vi "Arduino_I2CRead1.vi"() -> ()   [LabVIEW 2019]
uses:
  <vilib>/LabVIEW Interface for Arduino/LabVIEW Interface for Arduino.lvlib
  <vilib>/LabVIEW Interface for Arduino/Type Defs/Connection Type.ctl
  <vilib>/LabVIEW Interface for Arduino/Type Defs/Board Type.ctl
panel:
  out "Erro I2C Write":errorcluster
  out "error out":errorcluster
  out "I2C Data":u8[](array[numeric])
  out "?":dbl
  out "Signal":waveform(dbl)(graph)
  in  "Stopp":bool
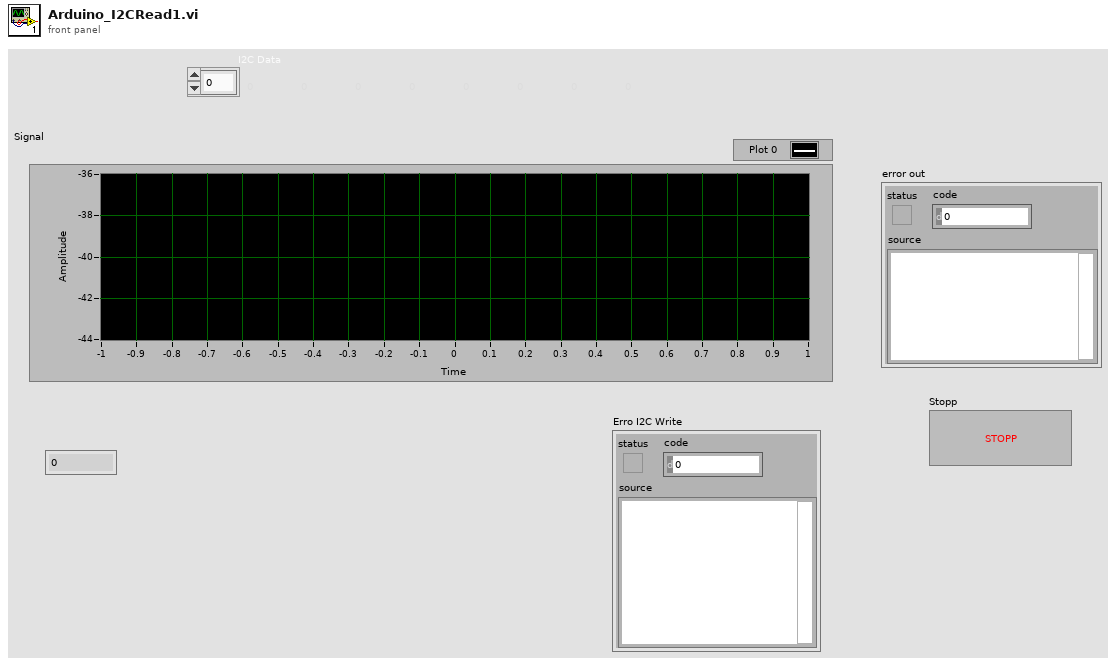
[diagram p1: front panel]
types:
  T1 = typedef "LabVIEW Interface for Arduino.lvlib/Board Type.ctl" = enum16{"Uno", "Dimuelanove w/Atmega 328", "Mega 2560"}
  T2 = typedef "LabVIEW Interface for Arduino.lvlib/Connection Type.ctl" = enum8{"USB / Serial", "XBEE", "BlueSmirf (Bluetooth)"}
  T3 = typedef "LabVIEW Interface for Arduino.lvlib/Arduino Resource.ctl" = cluster{"VISA resource":refnum<visa-resource-name>, "Board Type":T1, "Connection Type":enum8{"USB / Serial"}, "Bytes Per Packet (15)":u8}
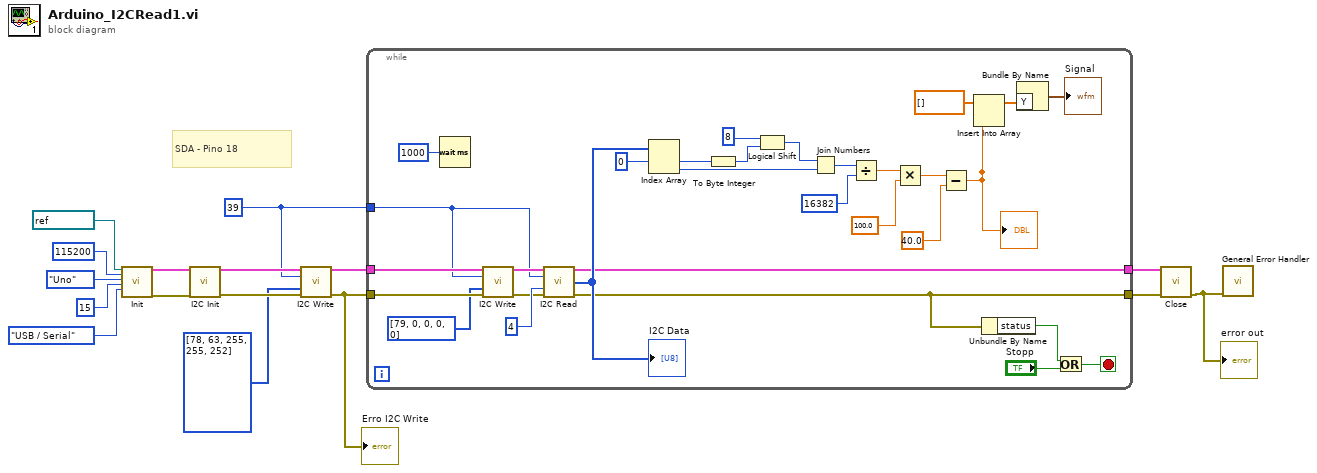
[diagram p0: block diagram]
diagram:
  w3 = u8 39 ("Address (0)")
  # "SDA - Pino 18"
  n1 = call <vilib>:"Init.vi"("VISA resource"=refnum<visa-resource-name> "COM3", "Baud Rate (115200)"=u32 115200, "Board Type (Uno)"=Board_Type."Uno", "Bytes Per Packet (15)"=u32 15, "Connection Type (USB/Serial)"=Connection_Type."USB / Serial") -> ("Arduino Resource"=w16:T3, "error out"=w15:errorcluster)  [unwired: 13 in]
  n2 = call <vilib>:"I2C Init.vi"("Arduino Resource"=w16, "error in"=w15) -> ("Arduino Resource"=w6:T3, "error out"=w4:errorcluster)  [unwired: 12 in]
  n3 = call <vilib>:"I2C Write.vi"("Arduino Resource"=w6, "Address (0)"=w3, "I2C Data Bytes"=u8[] [78, 63, 255, 255, 252] ("Data"), "error in"=w4) -> ("Arduino Resource"=w5:T3, "error out"=w1:errorcluster)  [unwired: 10 in]
  "Erro I2C Write" <- w1
  n4 = while {
    tunnel: w5 -> [w32]
    tunnel: w1 -> [w29]
    tunnel: [w24] -> w9
    tunnel: [w33] -> w7
    tunnel: w3 -> [w27]
    stop <- w41 stop-if-true
    n5 = Wait (ms)(milliseconds to wait=u32 1000 ("Zu wartende ms")) -> ()  [unwired: 1 out]
    n6 = call <vilib>:"I2C Write.vi"("Arduino Resource"=w32, "Address (0)"=w27, "I2C Data Bytes"=u8[] [79, 0, 0, 0, 0] ("Data"), "error in"=w29) -> ("Arduino Resource"=w31:T3, "error out"=w30:errorcluster)  [unwired: 10 in]
    n7 = call <vilib>:"I2C Read.vi"("Arduino Resource"=w31, "Address (0)"=w27, "Bytes To Read"=u8 4, "error in"=w30) -> ("Arduino Resource"=w33:T3, "I2C Data"=w40:u8[], "error out"=w24:errorcluster)  [unwired: 9 in]
    "I2C Data" <- w40
    n8 = Index Array(array=w40, index #1=0 ("Index")) -> (element #1=w23:u8, element #2=w21:u8)  [unwired: 1 in]
    n9 = To Byte Integer(number=w23) -> (8bit integer=w25:i8)
    n10 = Logical Shift(y=i16 8, x=w25) -> (x << y=w22:i8)
    n11 = Join Numbers(hi=w22, lo=w21) -> ((hi.lo)=w34:u16)
    n12 = Divide(x=w34, y=u16 16382) -> (x/y=w39:dbl)
    n13 = Multiply(x=w39, y=100.0) -> (x*y=w37:dbl)
    n14 = Subtract(x=w37, y=40.0) -> (x-y=w19:dbl)
    "?" <- w19
    n15 = Insert Into Array(array=dbl[] [], new element=w19) -> (w18:dbl[])  [unwired: 1 in]
    n16 = Unbundle By Name(w24) -> ("status"=w43:bool)
    n17 = Bundle By Name("Y"=w18) -> (→"Signal":waveform(dbl))  [unwired: 1 in]
    n18 = Or(x=w43, y="Stopp") -> (x .or. y?=w41:bool)
  }
  n19 = call <vilib>:"Close.vi"("Arduino Resource"=w7, "error in"=w9) -> ("error out"=w8:errorcluster)  [unwired: 13 in]
  "error out" <- w8
  n20 = call <vilib>:"General Error Handler.vi"("error in (no error)"=w8) -> ()  [unwired: 10 in, 5 out]
